vi "Get Item by name.vi"(8 "error in (no error)":errorcluster, 10 "name":string, 11 "JSON Object in":refnum<class "JSON Object.lvclass">) -> (0 "error out":errorcluster, 1 "found":bool, 2 "Value":refnum<class "JSON Value.lvclass">, 3 "JSON Object out":refnum<class "JSON Object.lvclass">)   [LabVIEW 2020, in "Library Commun.lvlib" / "JSON Object.lvclass"]
uses:
  JSON Object.lvclass
  JSON Value/JSON Value.lvclass
  JSON Object.lvclass/JSON Object.ctl
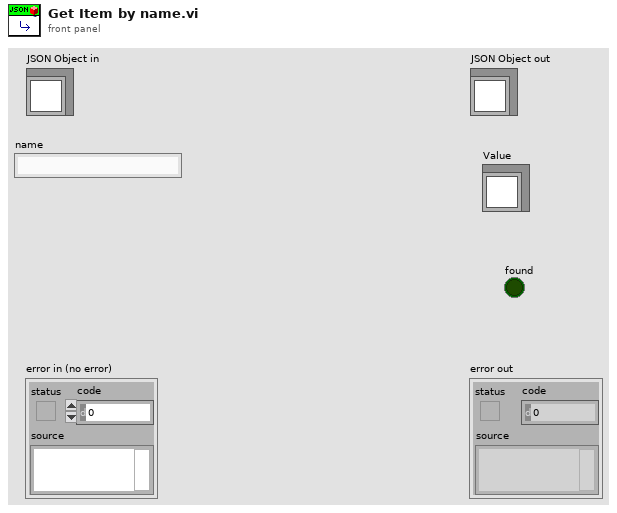
[diagram p1: front panel]
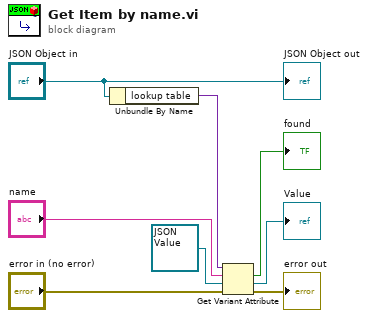
[diagram p0: block diagram]
diagram:
  n1 = Unbundle By Name("JSON Object in") -> ("lookup table"=w7:variant)
  n2 = Get Variant Attribute(Variant=w7, name="name", default value (empty Variant)=refnum<class "JSON Value.lvclass"> refnum ("JSON Value.lvclass"), error in="error in (no error)") -> (found=→"found":bool, value=→"Value":refnum<class "JSON Value.lvclass">, error out=→"error out":errorcluster)  [unwired: 1 out]
  "JSON Object out" <- "JSON Object in"
